vi "INTELLIFAUCET DO Control.vi"(0 "VISA session":refnum<visa-resource-name>="MW100", 1 "Normally Closed Valve?":bool, 5 "HEWH MW100 Channel Numbers":T3="011", 7 "Normally Closed Valve":T2, 9 "Normally Open Valve":T1, 11 "Error In":errorcluster) -> (4 "dup VISA session":refnum<visa-resource-name>, 6 "Power ON":bool, 8 "Message":string, 15 "error out":errorcluster)   [LabVIEW 2016]
uses:
  MW100/Type Definitions/HEWH MW100 Channel Numbers.ctl
  Type Definitions/HEWH Normally Closed Valve Control.ctl
  Type Definitions/HEWH Normally Open Valve Control.ctl
panel:
  # "PWR_MAIN: CLOSED = POWER OFF"
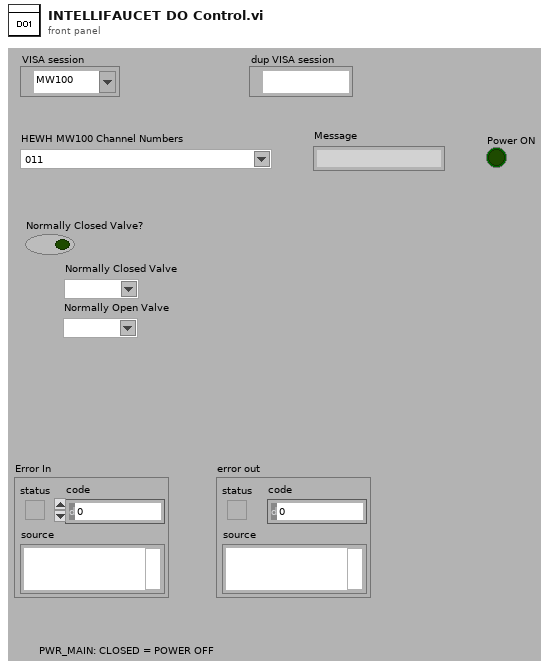
[diagram p1: front panel]
types:
  T1 = typedef "HEWH Normally Open Valve Control.ctl" = string
  T2 = typedef "HEWH Normally Closed Valve Control.ctl" = string
  T3 = typedef "HEWH MW100 Channel Numbers.ctl" = string
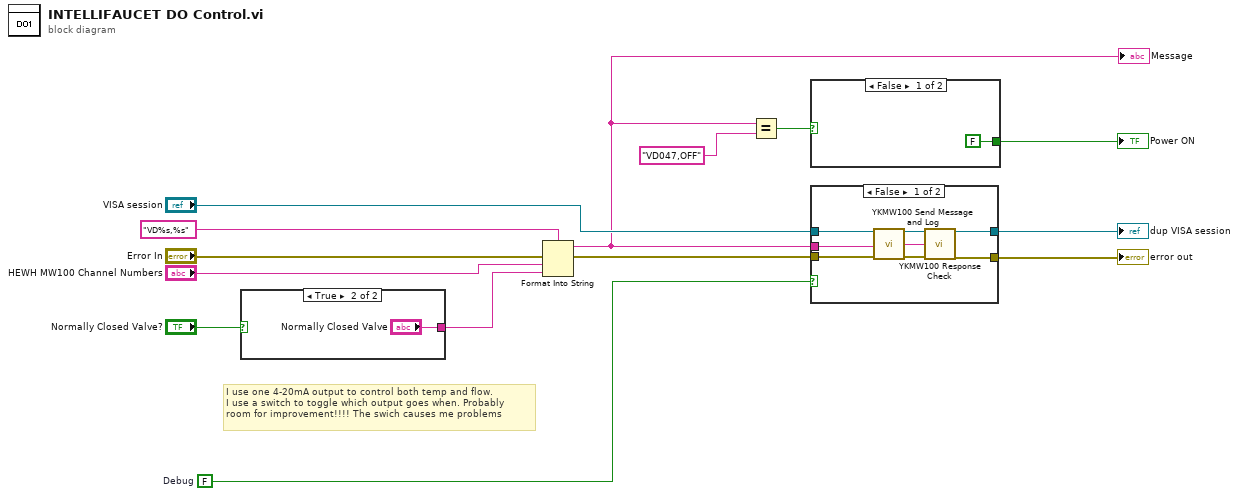
[diagram p0: block diagram]
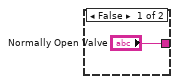
[diagram p2: hidden frame]
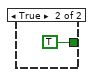
[diagram p4: hidden frame]
diagram:
  w3 = FALSE  # Debug
  # "I use one 4-20mA output to control both temp and flow.\nI use a switch to toggle which output goes when. Probably\nroom for improvement!!!! The swich causes me problems"
  n1 = case shown="True" "Normally Closed Valve?" {
    tunnel: ["Normally Open Valve" "Normally Closed Valve"] -> w2
    frame False {
    }
    frame True {
    }
  }
  n2 = Format Into String(format string="VD%s,%s", error in="Error In", "HEWH MW100 Channel Numbers", w2) -> (resulting string=w6:string, error out=w10:errorcluster)  [unwired: 1 in]
  "Message" <- w6
  n3 = Equal?(x=w6, y="VD047,OFF") -> (x = y?=w7:bool)
  n4 = case shown="False" w7 {
    tunnel: [FALSE TRUE] -> w4
    frame False {
    }
    frame True {
    }
  }
  "Power ON" <- w4
  n5 = case shown="False" w3 {
    tunnel: "VISA session" -> [w26 w27]
    tunnel: [w25 w27] -> w13
    tunnel: [w24 w28] -> w12
    tunnel: w10 -> [w23 w28]
    tunnel: w6 -> [w19 _]
    frame False {
      n6 = call "YKMW100 Send Message and Log.vi"("VISA session"=w26, "Send Message (\"\")"=w19, "error in (no error)"=w23) -> ("dup VISA session"=w22:refnum<visa-resource-name>, "Read Buffer"=w20:string, "error out"=w21:errorcluster)  [unwired: 10 in]
      n7 = call "YKMW100 Response Check.vi"("VISA session"=w22, "Message In (\"\")"=w20, "error in (no error)"=w21) -> ("dup VISA session"=w25:refnum<visa-resource-name>, "error out"=w24:errorcluster)  [unwired: 8 in, 3 out]
    }
    frame True {
    }
  }
  "dup VISA session" <- w13
  "error out" <- w12
